vi "Read stop loops flag.vi"(8 "error in (no error)":errorcluster) -> (0 "error out":errorcluster, 3 "Stop all loops?":bool)   [LabVIEW 2020, in "global_stop_flag.lvlib"]
uses:
  global_stop_flag.lvlib
  Stop Loops--Global Variable.vi
panel:
  # "Development\ncontrols/indicators useful for development and testing, but which are not outputs of the VI"
  # "Input\nInputs to the VI"
  # "Output\nOutputs of the VI"
  # "Description\n\nBlank VI with error handling case. \n\nSummarize the use of this VI in this space."
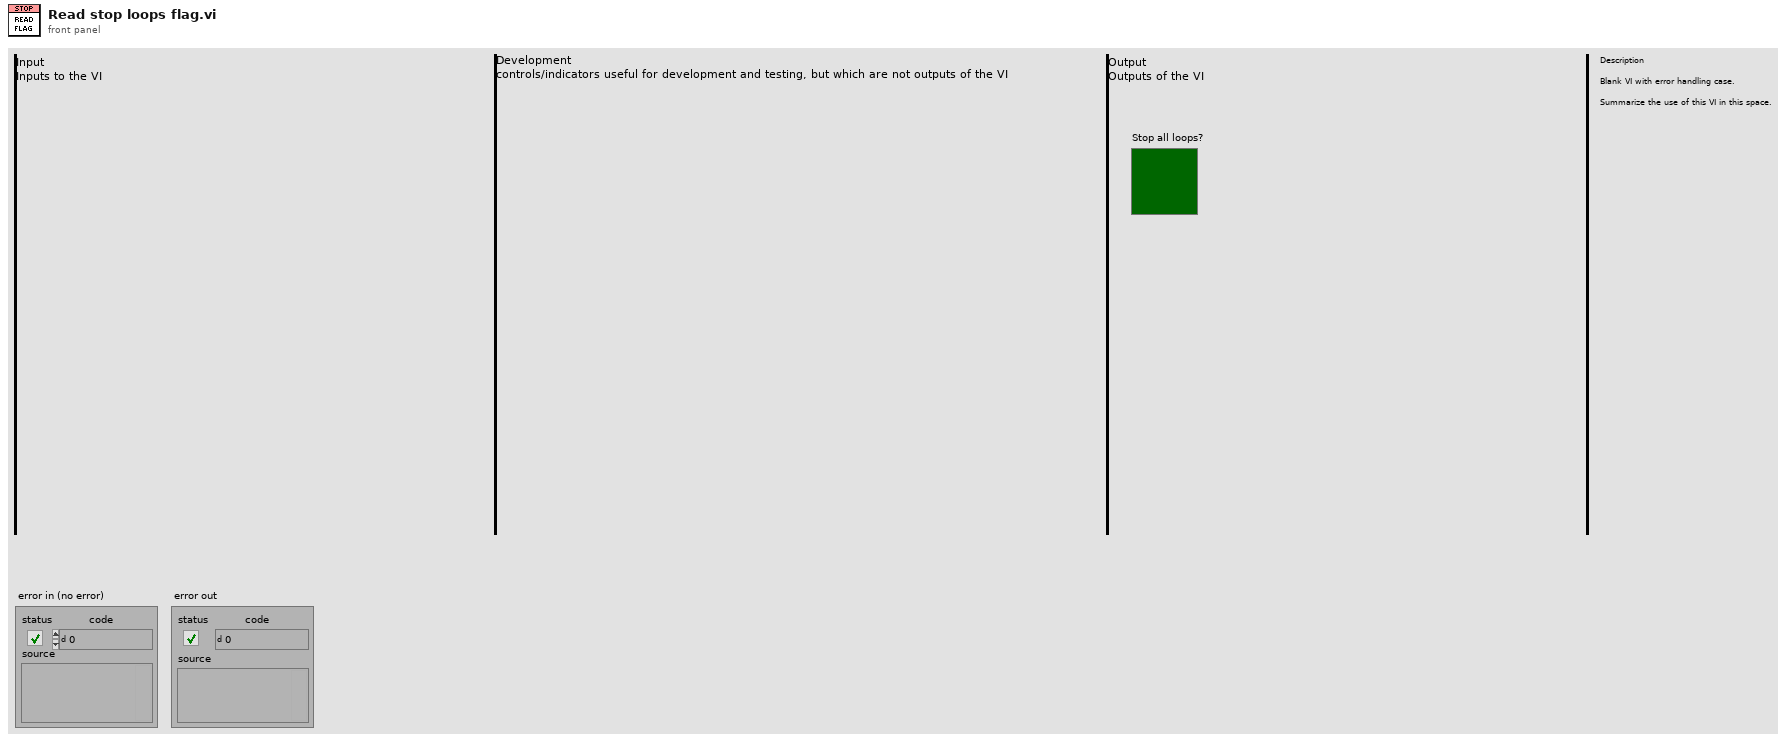
[diagram p1: front panel]
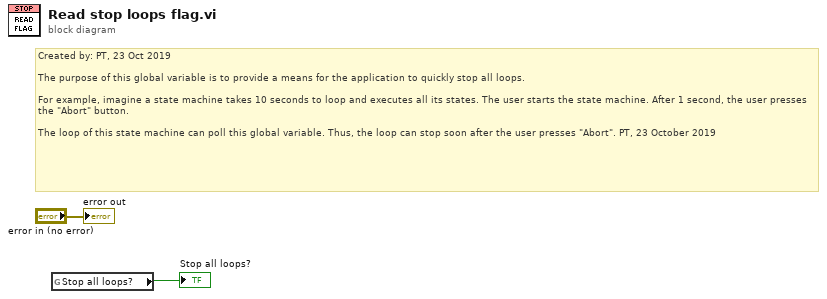
[diagram p0: block diagram]
diagram:
  # "Created by: PT, 23 Oct 2019\n\nThe purpose of this global variable is to provide a means for the application to quickly stop all loops.\n\nFor example, imagine a state machine takes 10 seconds to loop and executes all its states. The user starts the state machine. After 1 second, the user presses the \"Abort\" button.\n\nThe loop of this state machine can poll this global variable. Thus, the loop can stop soon after the user presses \"Abort\". PT, 23 October 2019"
  n1 = global read "Stop Loops--Global Variable.vi" "Stop all loops?"() -> (→"Stop all loops?":bool)
  "error out" <- "error in (no error)"
